vi "Do.vi"(8 "error in (no error)":errorcluster, 10 "queue out":refnum<queue>, 11 "State Cmd in":refnum<class "Message.lvclass">) -> (0 "error out":errorcluster, 3 "State Cmd out":refnum<class "Message.lvclass">)   [LabVIEW 2020, in "OOP SM.lvlib" / "Message.lvclass"]
uses:
  Message.lvclass
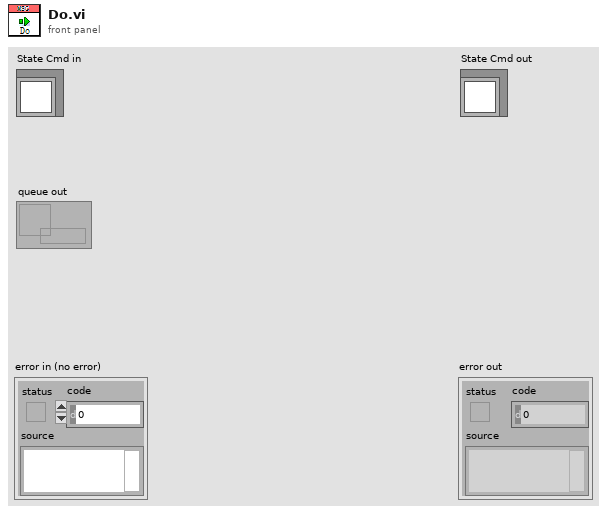
[diagram p1: front panel]
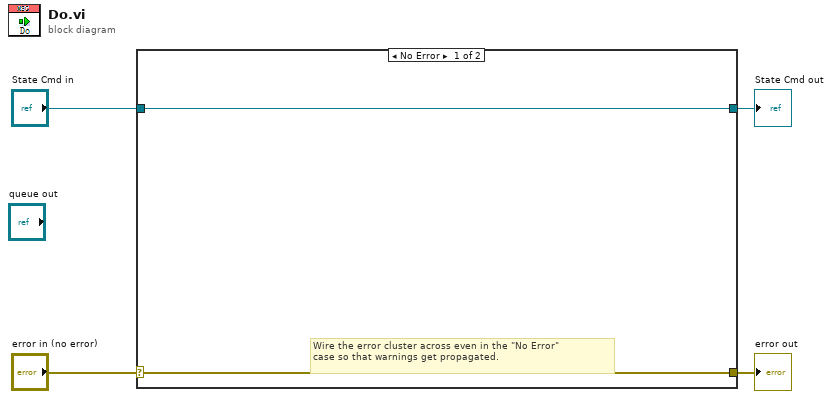
[diagram p0: block diagram]
diagram:
  n1 = case shown="No Error" "error in (no error)" {
    selector: "error in (no error)" -> [w5 w8]
    tunnel: [w5 w8] -> w3
    tunnel: [w6 w7] -> w1
    tunnel: "State Cmd in" -> [w6 w7]
    frame No Error {
      # "Wire the error cluster across even in the \"No Error\"\ncase so that warnings get propagated."
    }
    frame Error {
    }
  }
  "error out" <- w3
  "State Cmd out" <- w1
